vi "Multi-Channel ADC Viewer.vi"(0 "Channel Selection":T4, 1 "Start":bool, 5 "ADC Type":T1={"Channel Type"=enum."Single", "Resolution"=enum."8"}, 9 "Stop":bool, 11 "error in":errorcluster) -> (4 "Digital Waveform Graph":digitalwaveform(graph), 15 "error out":errorcluster)   [LabVIEW 2023]
doc: "This is simple ADC viewer which can plot the ADC data from the Analog to Digital conversion VI of different channels based on the user input, It can be a single channel viewer or a multi channel viewer. User can configure the resolution of the ADC. And also desired channels can be selected to view the ADC waveform."
uses:
  Type def/ChannelSelection.ctl
  Type def/ADCType.ctl
  Type def/ChannelType.ctl
  Type def/Resolution.ctl
  Type def/QueueOperations.ctl
  Type def/variant.ctl
  Type def/DataCluster.ctl
  Classes/Model Driver/Model Driver.lvclass
  Type def/U8ArrayCluster.ctl
panel:
  in  "Reset":bool
  # "MULTI-CHANNEL ADC VIEWER"
  # "INSTRUCTIONS\n\n1. Run the VI.\n2. Select the ADC Type -> Channel Type and Resolution.\n3. Channel Type can be -> Single Channel or 4-Channel.\n4. Resolution can be -> 2,4,8,12 or 16 bits.\n5. Use Channel selection option to view a particular channel\n    when using 4-Channel ADC.\n5. Press Start to start the ADC.\n6. Press Stop to stop the ADC.\n7. Press Reset to clear the Waveform Graph.\n8. Panel Close to Abort the VI."
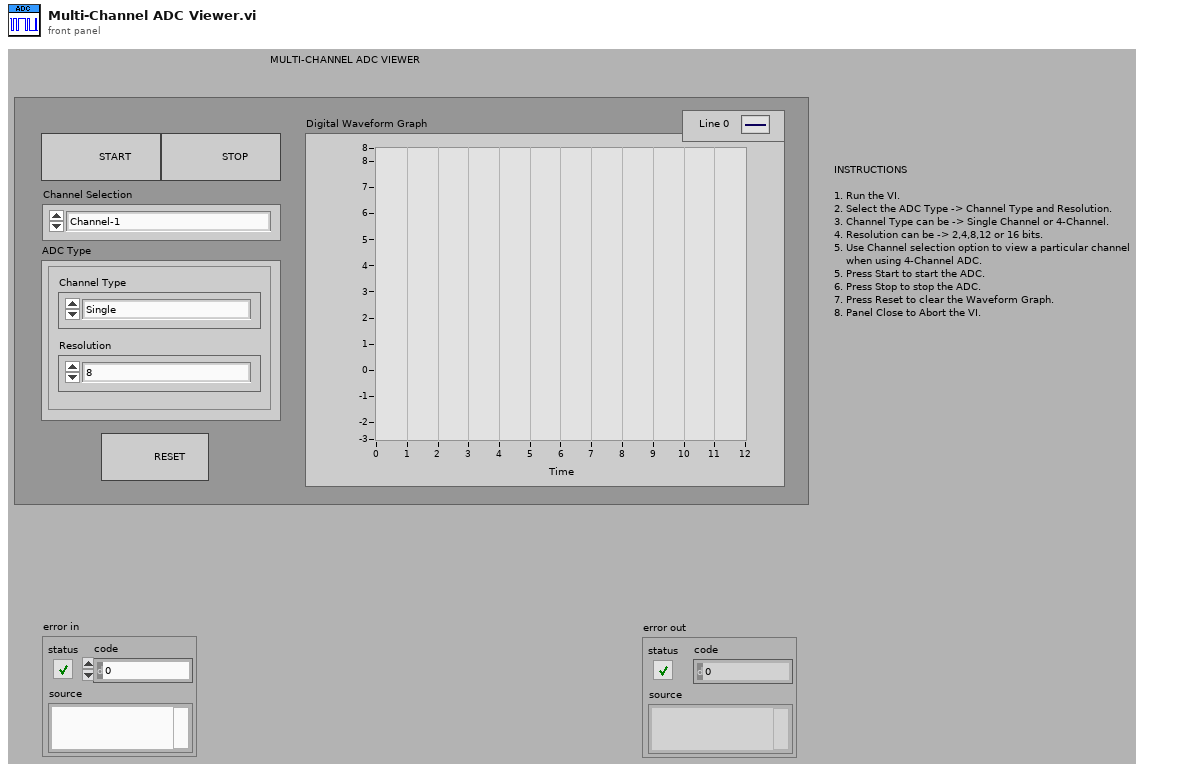
[diagram p1: front panel]
types:
  T1 = typedef "ADCType.ctl" = cluster{"Channel Type":T2, "Resolution":T3}
  T2 = typedef "ChannelType.ctl" = enum16{"Single", "4-Channel"}
  T3 = typedef "Resolution.ctl" = enum16{"2", "4", "8", "12", "16"}
  T4 = typedef "ChannelSelection.ctl" = enum16{"Channel-1", "Channel-2", "Channel-3", "Channel-4"}
  T5 = typedef "DataCluster.ctl" = cluster{"Stop":bool, "File Path":path, "Channel Selection":T4, "ADC Type":T1, "Digital Waveform Graph":digitalwaveform, "Start Time":dbl, "Elapsed Time":dbl, "Start":bool, "Model Driver Class":refnum<class "Model Driver.lvclass">, "Stop User Event":refnum<user-event>, "U8 Arrays":T6}
  T6 = typedef "U8ArrayCluster.ctl" = cluster{"Single Channel U8 array":u8[], "Mult Channel U8 array":u8[][], "1D Multi Channel U8 Array":u8[], "Channel 1 U8 Array":u8[], "Channel 2 U8 Array":u8[], "Channel 3 U8 Array":u8[], "Channel 4 U8 Array":u8[]}
  T7 = typedef "variant.ctl" = cluster{"Data":variant, "State":string}
  T8 = typedef "QueueOperations.ctl" = enum16{"Create", "Enqueue", "Enqueue N elements", "Dequeue", "Flush", "Release"}
  T9 = enum8{"Enabled", "Disabled", "Disabled and Grayed Out"}
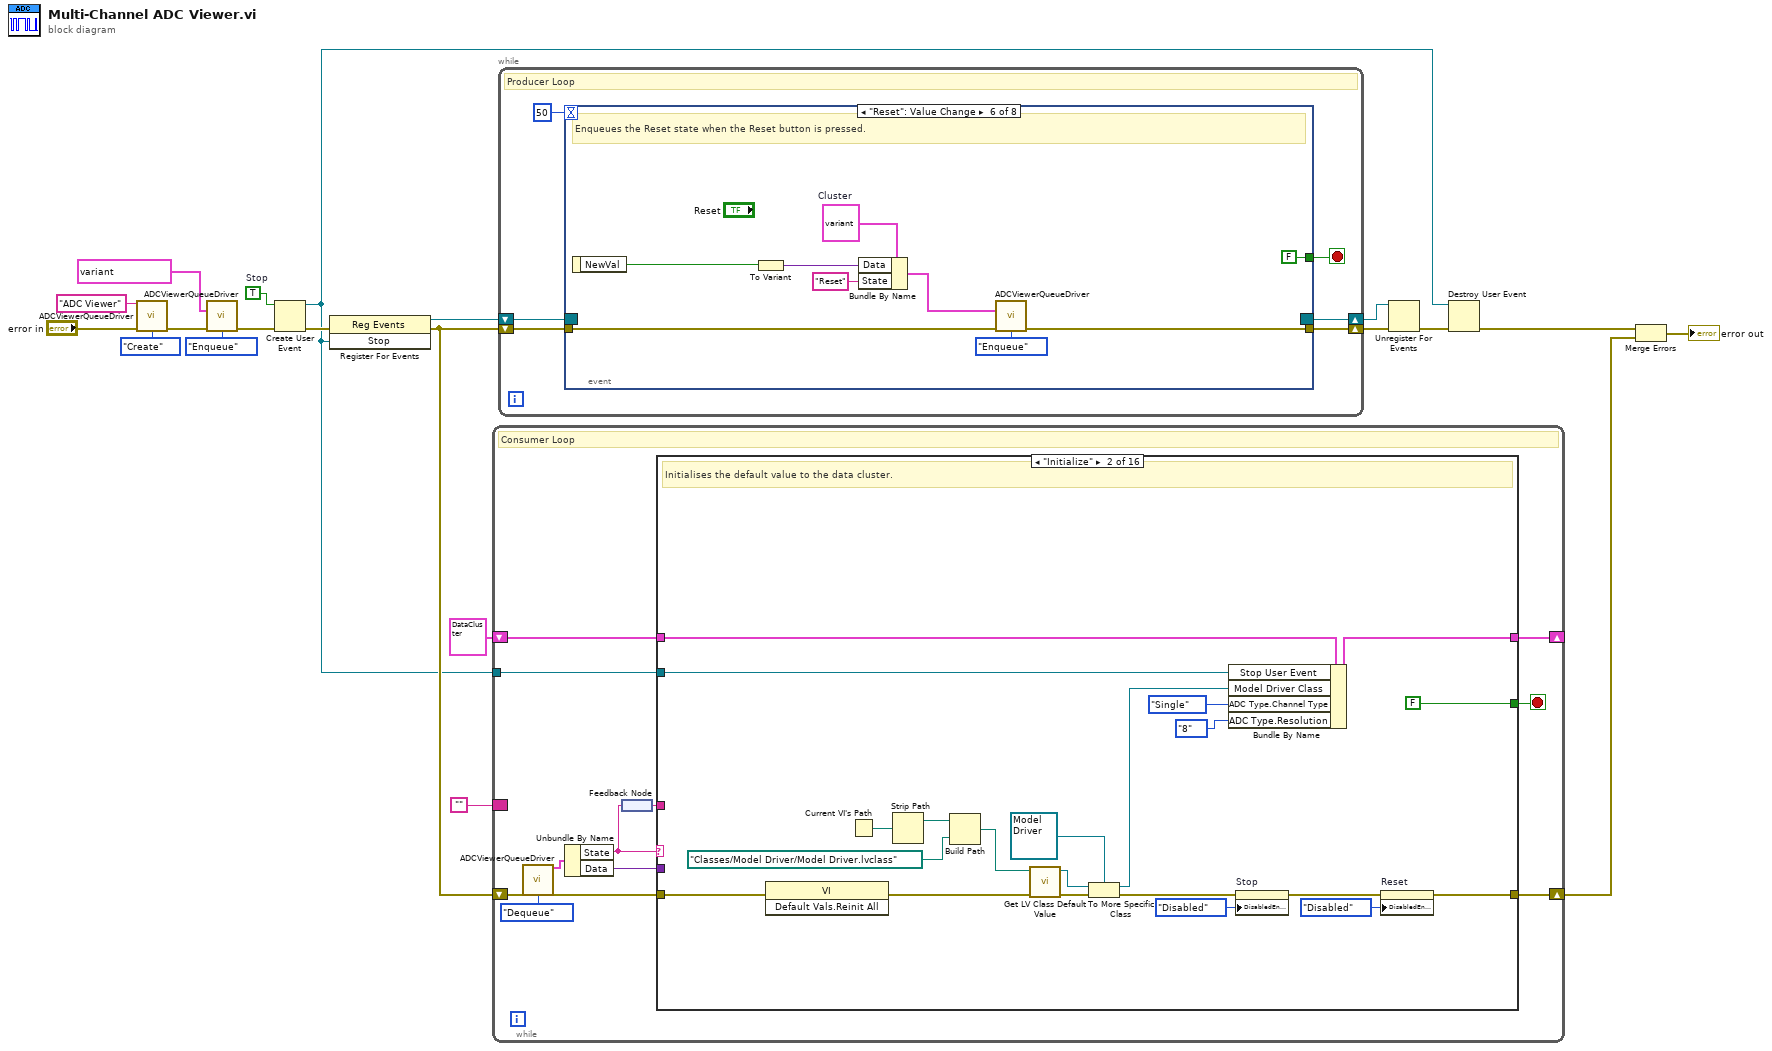
[diagram p0: block diagram]
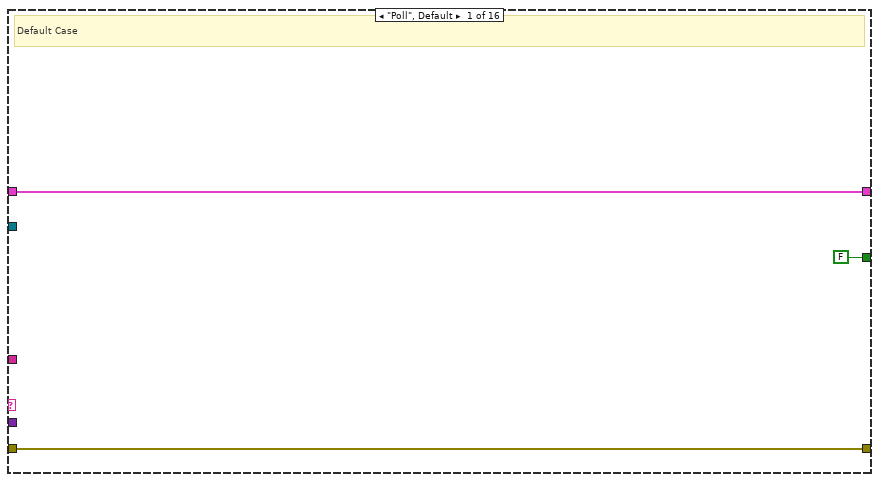
[diagram p2: hidden frame]
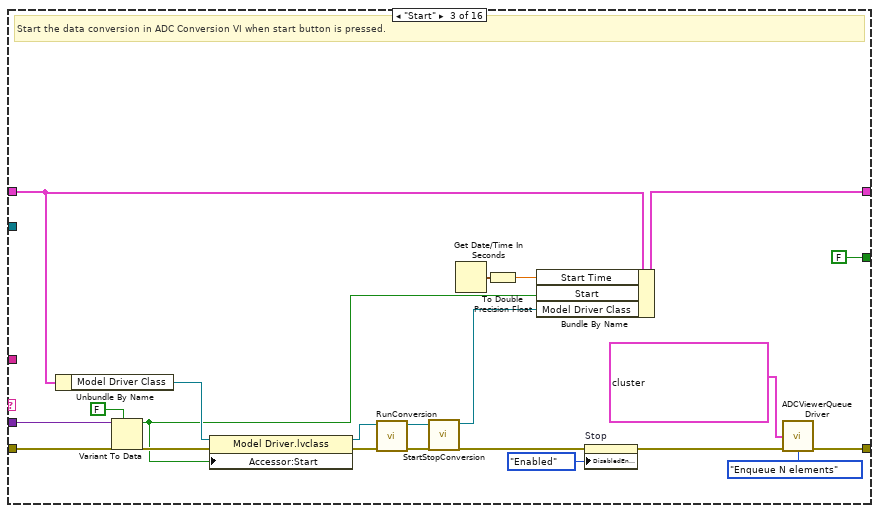
[diagram p3: hidden frame]
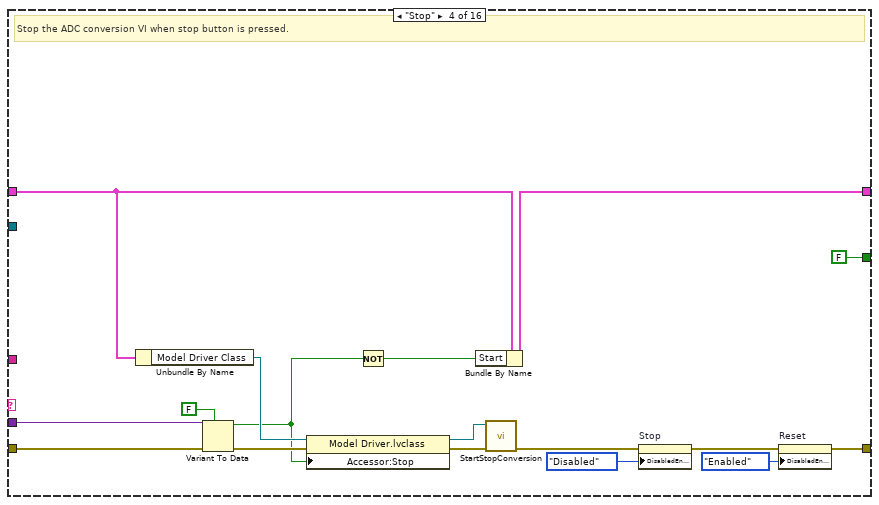
[diagram p4: hidden frame]
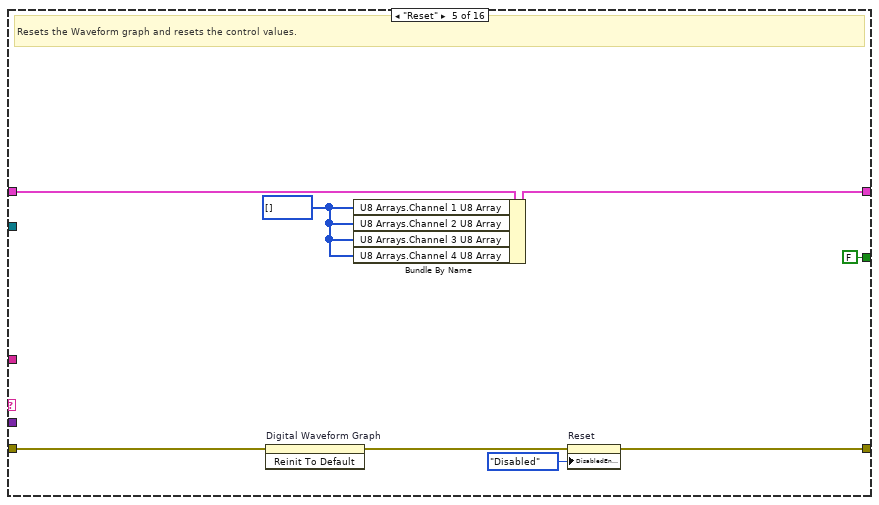
[diagram p5: hidden frame]
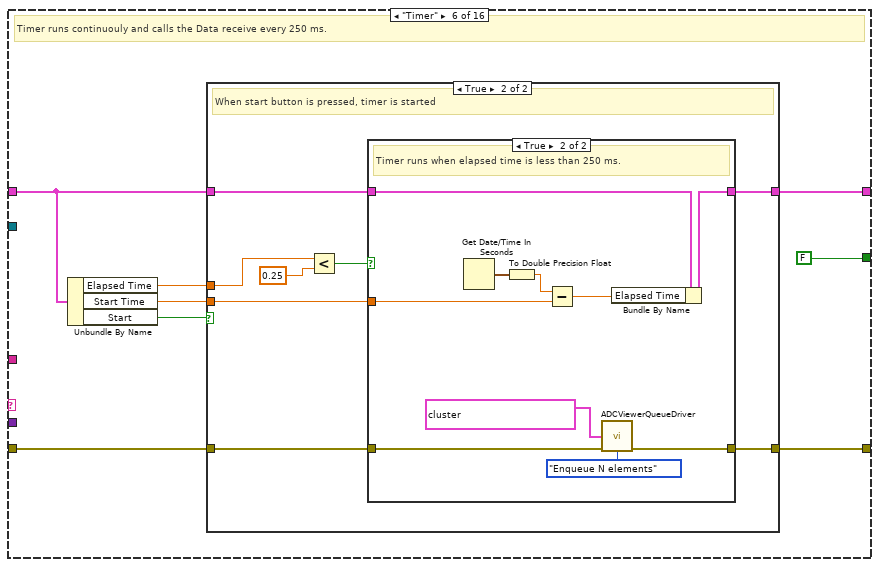
[diagram p6: hidden frame]
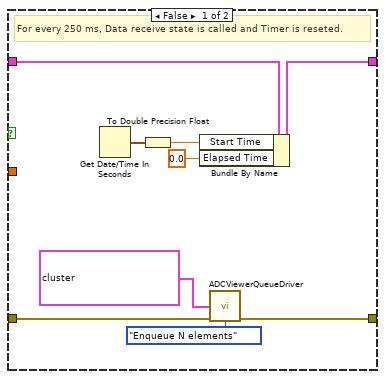
[diagram p8: hidden frame]
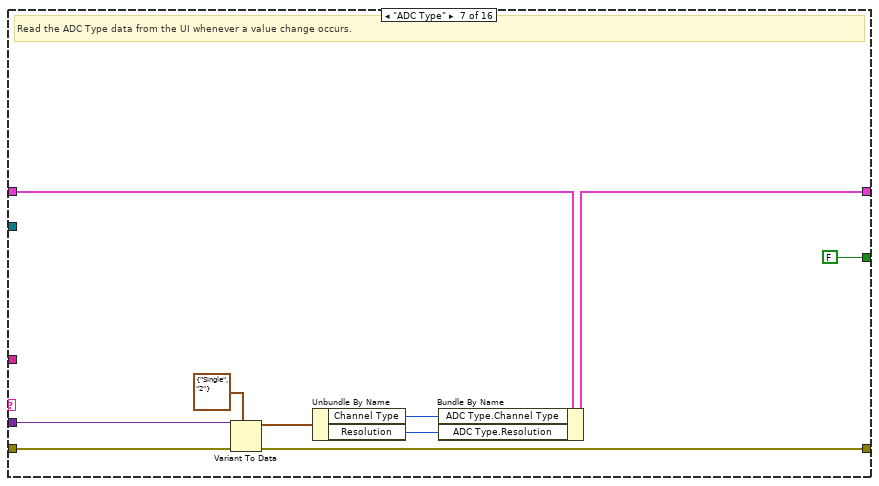
[diagram p9: hidden frame]
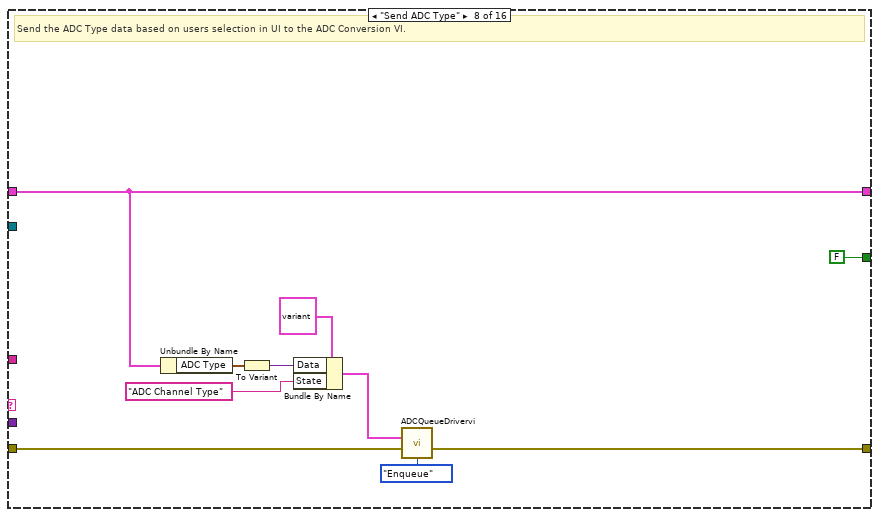
[diagram p10: hidden frame]
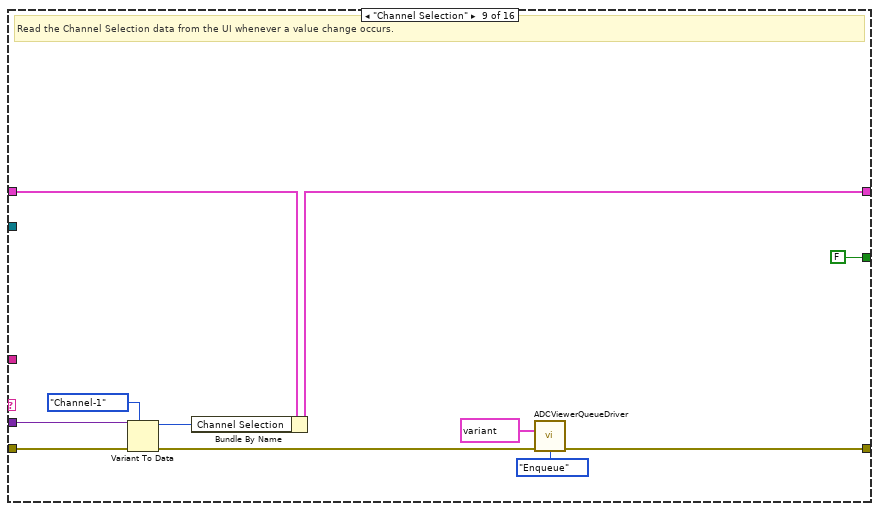
[diagram p11: hidden frame]
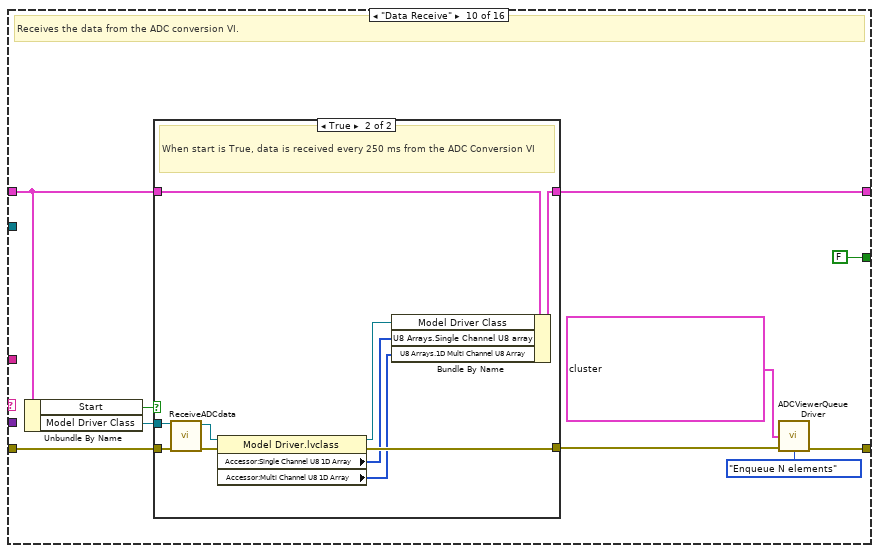
[diagram p12: hidden frame]
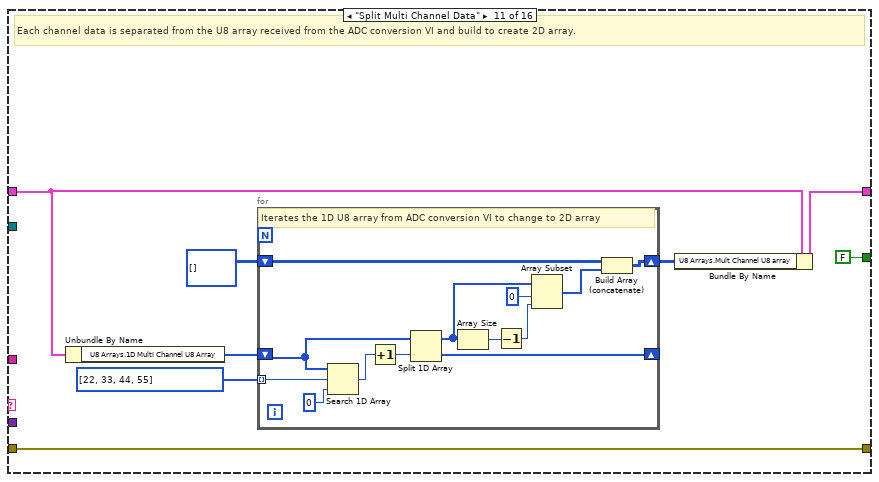
[diagram p14: hidden frame]
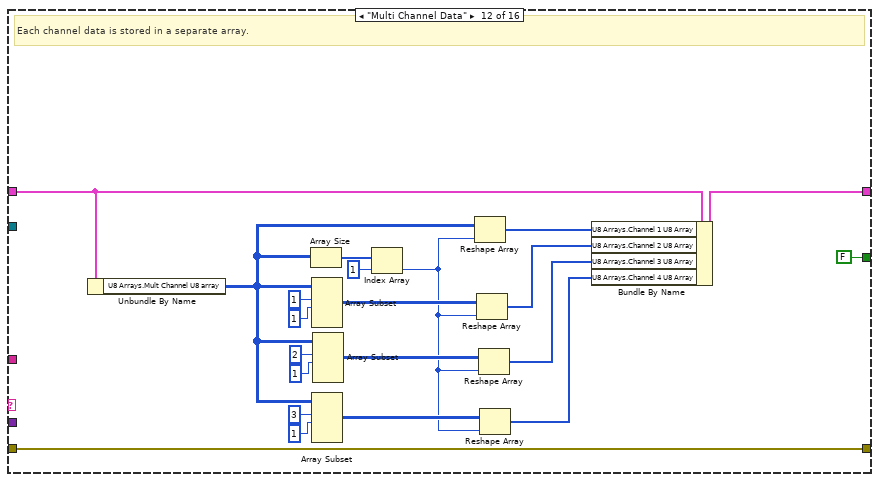
[diagram p15: hidden frame]
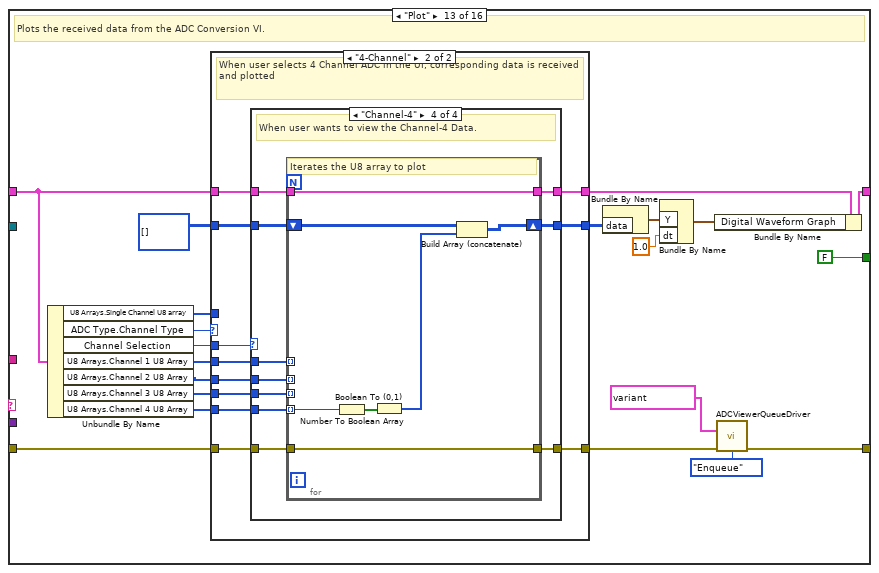
[diagram p16: hidden frame]
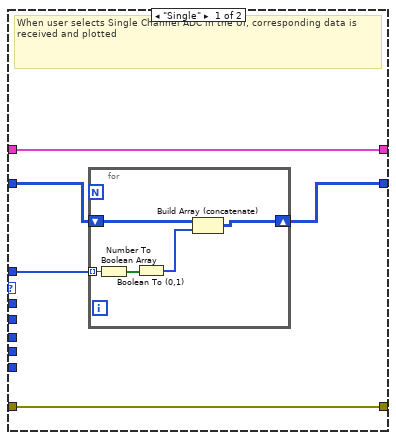
[diagram p17: hidden frame]
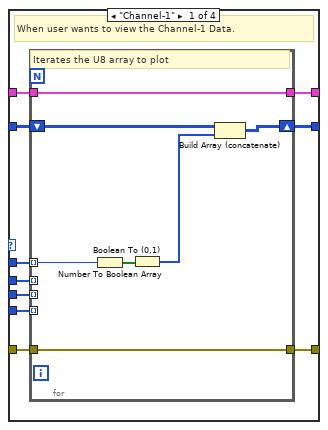
[diagram p18: hidden frame]
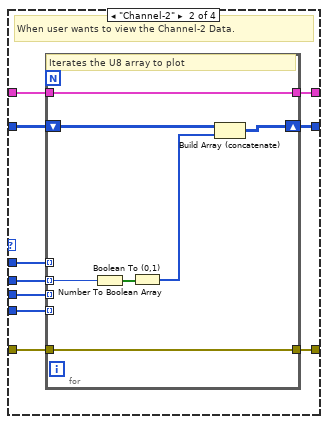
[diagram p19: hidden frame]
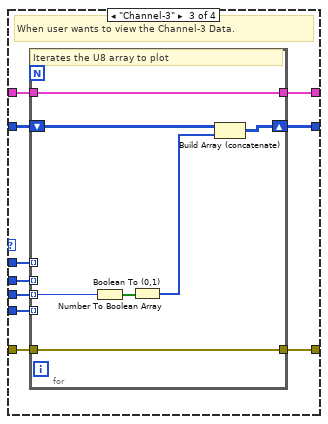
[diagram p20: hidden frame]
diagram:
  w8 = TRUE  # Stop
  n1 = call "ADCViewerQueueDriver.vi"("Queue Name"="ADC Viewer", "error in"="error in", "Queue Operations"=QueueOperations."Create") -> ("error out"=w19:errorcluster)  [unwired: 11 in, 1 out]
  n2 = call "ADCViewerQueueDriver.vi"("Enqueue State"=T7 {"Data"=variant, "State"="Initialize"}, "error in"=w19, "Queue Operations"=QueueOperations."Enqueue") -> ("error out"=w18:errorcluster)  [unwired: 11 in, 1 out]
  n3 = Create User Event(user event datatype=w8, error in=w18) -> (user event=w1:refnum<user-event>, error out=w9:errorcluster)
  n4 = register-events(error in=w9, w1) -> (reference out=w6:refnum<event-registration>, error out=w7:errorcluster)  [unwired: 1 in]
  n5 = while {
    shift-right: [w32] -> w13
    shift-left: w7 -> [w31]
    shift-right: [w24] -> _
    shift-left: T5 {"Stop"=FALSE, "File Path"=path "", "Channel Selection"=enum."Channel-1", "ADC Type"={"Channel Type"=enum."Single", "Resolution"=enum."2"}, "Digital Waveform Graph"={"t0"=timestamp(0 s since 1904-01-01), "dt"=0.0, "Y"={"transitions"=[], "data"=[]}}, "Start Time"=0.0, "Elapsed Time"=0.0, "Start"=FALSE, "Model Driver Class"=refnum, "Stop User Event"=refnum, "U8 Arrays"={"Single Channel U8 array"=[], "Mult Channel U8 array"=[], "1D Multi Channel U8 Array"=[], "Channel 1 U8 Array"=[], "Channel 2 U8 Array"=[], "Channel 3 U8 Array"=[], "Channel 4 U8 Array"=[]}} ("Cluster") -> [w25]
    border: "" -> [_]
    tunnel: w1 -> [w21]
    stop <- w26 stop-if-true
    # "Consumer Loop"
    n6 = call "ADCViewerQueueDriver.vi"("error in"=w31, "Queue Operations"=QueueOperations."Dequeue") -> ("Dequeue State"=w29:T7, "error out"=w30:errorcluster)  [unwired: 12 in]
    n7 = Unbundle By Name(w29) -> ("State"=w23:string, "Data"=w28:variant)
    n8 = feedback-in #1(w23) -> ()
    n9 = feedback #1() -> (w22:string)
    n10 = case shown="\"Initialize\"" w23 {
      tunnel: w30 -> [w33 w56 w75 w93 w97 w106 w150 w158 w171 w181 w201 w235 w248 w349 w363 w377]
      tunnel: [w33 w46 w70 w81 w100 w105 w141 w157 w162 w178 w201 w235 w238 w349 w353 w381] -> w32
      tunnel: w28 -> [_ _ w74 w92 _ _ w142 _ w167 _ _ _ _ _ _ _]
      tunnel: [FALSE FALSE FALSE FALSE FALSE FALSE FALSE FALSE FALSE FALSE FALSE FALSE FALSE FALSE FALSE TRUE] -> w26
      tunnel: w25 -> [w34 w54 w67 w89 w103 w110 w149 w156 w170 w175 w197 w234 w251 w347 w351 w383]
      tunnel: [w34 w50 w72 w91 w99 w109 w147 w156 w169 w179 w198 w219 w241 w347 w351 w383] -> w24
      tunnel: w22 -> [_ _ _ _ _ _ _ _ _ _ _ _ _ _ w362 _]
      tunnel: w21 -> [_ w47 _ _ _ _ _ _ _ _ _ _ _ _ _ _]
      frame "Poll", Default {
        # "Default Case"
      }
      frame "Initialize" {
        # "Initialises the default value to the data cluster."
        n11 = invoke class="VI" method="Default Vals.Reinit All"(error in=w56) -> (error out=w53:errorcluster)  [unwired: 2 in, 2 out]
        n12 = Current VI's Path() -> (path=w44:path)
        n13 = Strip Path(path=w44) -> (stripped path=w43:path)  [unwired: 1 out]
        n14 = Build Path(base path=w43, name or relative path=path "Classes/Model Driver/Model Driver.lvclass") -> (appended path=w41:path)
        n15 = call <vilib>:"Get LV Class Default Value.vi"("error in (no error)"=w53, "class path"=w41) -> ("error out"=w52:errorcluster, "object"=w51:refnum<class>)  [unwired: 8 in]
        n16 = To More Specific Class(target class=refnum<class "Model Driver.lvclass"> refnum ("Model Driver.lvclass"), reference=w51, error in=w52) -> (specific class reference=w48:refnum<class "Model Driver.lvclass">, error out=w37:errorcluster)
        n17 = Bundle By Name(cluster=w54, "Stop User Event"=w47, "Model Driver Class"=w48, "ADC Type.Channel Type"=ChannelType."Single", "ADC Type.Resolution"=Resolution."8") -> (w50:T5)
        n18 = property on="Stop" class="Bool"(error in=w37, "DisabledEnum"=T9."Disabled" ("Disabled")) -> (error out=w36:errorcluster)  [unwired: 1 in, 1 out]
        n19 = property on="Reset" class="Bool"(error in=w36, "DisabledEnum"=T9."Disabled" ("Disabled")) -> (error out=w46:errorcluster)  [unwired: 1 in, 1 out]
      }
      frame "Start" {
        # "Start the data conversion in ADC Conversion VI when start button is pressed."
        n20 = Unbundle By Name(w67) -> ("Model Driver Class"=w66:refnum<class "Model Driver.lvclass">)
        n21 = Variant To Data(error in=w75, type=FALSE, Variant=w74) -> (data=w65:bool, error out=w69:errorcluster)
        n22 = property class="Model Driver.lvclass"(reference=w66, error in=w69, "Accessor:Start"=w65) -> (reference out=w64:refnum<class "Model Driver.lvclass">, error out=w63:errorcluster)
        n23 = call "RunConversion.vi"("error in (no error)"=w63, "Model Driver in"=w64) -> ("error out"=w61:errorcluster, "Model Driver out"=w62:refnum<class "Model Driver.lvclass">)  [unwired: 8 in]
        n24 = call "StartStopConversion.vi"("error in (no error)"=w61, "Model Driver in"=w62) -> ("error out"=w59:errorcluster, "Model Driver out"=w57:refnum<class "Model Driver.lvclass">)  [unwired: 8 in]
        n25 = Get Date/Time In Seconds() -> (seconds since 1Jan1904=w77:timestamp)
        n26 = To Double Precision Float(number=w77) -> (double precision float=w76:dbl)
        n27 = Bundle By Name(cluster=w67, "Start Time"=w76, "Start"=w65, "Model Driver Class"=w57) -> (w72:T5)
        n28 = property on="Stop" class="Bool"(error in=w59, "DisabledEnum"=T9."Enabled" ("Disabled")) -> (error out=w58:errorcluster)  [unwired: 1 in, 1 out]
        n29 = call "ADCViewerQueueDriver.vi"("Array State"=T7[] [{"Data"=variant, "State"="Send ADC Type"}, {"Data"=variant, "State"="Timer"}], "error in"=w58, "Queue Operations"=QueueOperations."Enqueue N elements") -> ("error out"=w70:errorcluster)  [unwired: 11 in, 1 out]
      }
      frame "Stop" {
        # "Stop the ADC conversion VI when stop button is pressed."
        n30 = Unbundle By Name(w89) -> ("Model Driver Class"=w88:refnum<class "Model Driver.lvclass">)
        n31 = Variant To Data(error in=w93, type=FALSE, Variant=w92) -> (data=w85:bool, error out=w87:errorcluster)
        n32 = property class="Model Driver.lvclass"(reference=w88, error in=w87, "Accessor:Stop"=w85) -> (reference out=w84:refnum<class "Model Driver.lvclass">, error out=w86:errorcluster)
        n33 = Not(x=w85) -> (.not. x?=w90:bool)
        n34 = Bundle By Name(cluster=w89, "Start"=w90) -> (w91:T5)
        n35 = call "StartStopConversion.vi"("error in (no error)"=w86, "Model Driver in"=w84) -> ("error out"=w83:errorcluster)  [unwired: 8 in, 1 out]
        n36 = property on="Stop" class="Bool"(error in=w83, "DisabledEnum"=T9."Disabled" ("Disabled")) -> (error out=w82:errorcluster)  [unwired: 1 in, 1 out]
        n37 = property on="Reset" class="Bool"(error in=w82, "DisabledEnum"=T9."Enabled" ("Disabled")) -> (error out=w81:errorcluster)  [unwired: 1 in, 1 out]
      }
      frame "Reset" {
        w98 = u8[] [] ("U8 Arrays.Channel 1 U8 Array")
        # "Resets the Waveform graph and resets the control values."
        n38 = invoke on="Digital Waveform Graph" class="DigitalGraph (strict)" method="Reinit To Default"(error in=w97) -> (error out=w96:errorcluster)  [unwired: 2 in, 2 out]
        n39 = Bundle By Name(cluster=w103, "U8 Arrays.Channel 1 U8 Array"=w98, "U8 Arrays.Channel 2 U8 Array"=w98, "U8 Arrays.Channel 3 U8 Array"=w98, "U8 Arrays.Channel 4 U8 Array"=w98) -> (w99:T5)
        n40 = property on="Reset" class="Bool"(error in=w96, "DisabledEnum"=T9."Disabled" ("Disabled")) -> (error out=w100:errorcluster)  [unwired: 1 in, 1 out]
      }
      frame "Timer" {
        # "Timer runs continuouly and calls the Data receive every 250 ms."
        n41 = Unbundle By Name(w110) -> ("Elapsed Time"=w108:dbl, "Start Time"=w107:dbl, "Start"=w104:bool)
        n42 = case shown="True" w104 {
          tunnel: w110 -> [w113 w121]
          tunnel: [w113 w120] -> w109
          tunnel: w108 -> [_ w118]
          tunnel: w107 -> [_ w116]
          tunnel: w106 -> [w112 w115]
          tunnel: [w112 w114] -> w105
          frame False {
            # "When start button is not pressed."
          }
          frame True {
            # "When start button is pressed, timer is started"
            n43 = Less?(x=w118, y=0.25) -> (x < y?=w119:bool)
            n44 = case shown="True" w119 {
              tunnel: w121 -> [w130 w140]
              tunnel: [w129 w139] -> w120
              tunnel: w116 -> [_ w136]
              tunnel: w115 -> [w125 w134]
              tunnel: [w123 w133] -> w114
              frame False {
                # "For every 250 ms, Data receive state is called and Timer is reseted."
                n45 = Get Date/Time In Seconds() -> (seconds since 1Jan1904=w127:timestamp)
                n46 = To Double Precision Float(number=w127) -> (double precision float=w126:dbl)
                n47 = Bundle By Name(cluster=w130, "Start Time"=w126, "Elapsed Time"=0.0) -> (w129:T5)
                n48 = call "ADCViewerQueueDriver.vi"("Array State"=T7[] [{"Data"=variant, "State"="Timer"}, {"Data"=variant, "State"="Data Receive"}], "error in"=w125, "Queue Operations"=QueueOperations."Enqueue N elements") -> ("error out"=w123:errorcluster)  [unwired: 11 in, 1 out]
              }
              frame True {
                # "Timer runs when elapsed time is less than 250 ms."
                n49 = Get Date/Time In Seconds() -> (seconds since 1Jan1904=w138:timestamp)
                n50 = To Double Precision Float(number=w138) -> (double precision float=w137:dbl)
                n51 = Subtract(x=w137, y=w136) -> (x-y=w135:dbl)
                n52 = call "ADCViewerQueueDriver.vi"("Array State"=T7[] [{"Data"=variant, "State"="Timer"}, {"Data"=variant, "State"=""}], "error in"=w134, "Queue Operations"=QueueOperations."Enqueue N elements") -> ("error out"=w133:errorcluster)  [unwired: 11 in, 1 out]
                n53 = Bundle By Name(cluster=w140, "Elapsed Time"=w135) -> (w139:T5)
              }
            }
          }
        }
      }
      frame "ADC Type" {
        # "Read the ADC Type data from the UI whenever a value change occurs."
        n54 = Variant To Data(error in=w150, type=T1 {"Channel Type"=enum."Single", "Resolution"=enum."2"} ("NewVal"), Variant=w142) -> (data=w143:T1, error out=w141:errorcluster)
        n55 = Unbundle By Name(w143) -> ("Channel Type"=w146:T2, "Resolution"=w145:T3)
        n56 = Bundle By Name(cluster=w149, "ADC Type.Channel Type"=w146, "ADC Type.Resolution"=w145) -> (w147:T5)
      }
      frame "Send ADC Type" {
        # "Send the ADC Type data based on users selection in UI to the ADC Conversion VI."
        n57 = Unbundle By Name(w156) -> ("ADC Type"=w154:T1)
        n58 = To Variant(anything=w154) -> (Variant=w151:variant)
        n59 = Bundle By Name(cluster=T7 {"Data"=variant, "State"=""} ("Enqueue State"), "Data"=w151, "State"="ADC Channel Type") -> (w153:T7)
        n60 = call "ADCQueueDrivervi.vi"("Enqueue State"=w153, "error in"=w158, "Queue Operations"=QueueOperations."Enqueue") -> ("error out"=w157:errorcluster)  [unwired: 11 in, 1 out]
      }
      frame "Channel Selection" {
        # "Read the Channel Selection data from the UI whenever a value change occurs."
        n61 = Variant To Data(error in=w171, type=ChannelSelection."Channel-1" ("NewVal"), Variant=w167) -> (data=w165:T4, error out=w163:errorcluster)
        n62 = Bundle By Name(cluster=w170, "Channel Selection"=w165) -> (w169:T5)
        n63 = call "ADCViewerQueueDriver.vi"("Enqueue State"=T7 {"Data"=variant, "State"="Plot"}, "error in"=w163, "Queue Operations"=QueueOperations."Enqueue") -> ("error out"=w162:errorcluster)  [unwired: 11 in, 1 out]
      }
      frame "Data Receive" {
        # "Receives the data from the ADC conversion VI."
        n64 = Unbundle By Name(w175) -> ("Start"=w174:bool, "Model Driver Class"=w172:refnum<class "Model Driver.lvclass">)
        n65 = case shown="True" w174 {
          tunnel: w181 -> [w182 w191]
          tunnel: [w183 w193] -> w179
          tunnel: [w182 w189] -> w176
          tunnel: w175 -> [w183 w192]
          tunnel: w172 -> [_ w185]
          frame False {
            # "When Start is not pressed."
          }
          frame True {
            # "When start is True, data is received every 250 ms from the ADC Conversion VI"
            n66 = call "ReceiveADCdata.vi"("error in (no error)"=w191, "Model Driver in"=w185) -> ("error out"=w190:errorcluster, "Model Driver out"=w188:refnum<class "Model Driver.lvclass">)  [unwired: 8 in]
            n67 = property class="Model Driver.lvclass"(reference=w188, error in=w190) -> (reference out=w184:refnum<class "Model Driver.lvclass">, error out=w189:errorcluster, "Accessor:Single Channel U8 1D Array"=w187:u8[], "Accessor:Multi Channel U8 1D Array"=w186:u8[])
            n68 = Bundle By Name(cluster=w192, "Model Driver Class"=w184, "U8 Arrays.Single Channel U8 array"=w187, "U8 Arrays.1D Multi Channel U8 Array"=w186) -> (w193:T5)
          }
        }
        n69 = call "ADCViewerQueueDriver.vi"("Array State"=T7[] [{"Data"=variant, "State"="Split Multi Channel Data"}, {"Data"=variant, "State"="Multi Channel Data"}, {"Data"=variant, "State"="Plot"}], "error in"=w176, "Queue Operations"=QueueOperations."Enqueue N elements") -> ("error out"=w178:errorcluster)  [unwired: 11 in, 1 out]
      }
      frame "Split Multi Channel Data" {
        # "Each channel data is separated from the U8 array received from the ADC conversion VI and build to create 2D array."
        n70 = Unbundle By Name(w197) -> ("U8 Arrays.1D Multi Channel U8 Array"=w194:u8[])
        n71 = for {
          shift-right: [w204] -> _
          shift-left: w194 -> [w211]
          tunnel: u8[] [22, 33, 44, 55] ("array") -> [w210] mode=indexing
          shift-right: [w202] -> w196
          shift-left: u8[][] [] ("subarray") -> [w206]
          # "Iterates the 1D U8 array from ADC conversion VI to change to 2D array"
          n72 = Search 1D Array(1D array=w211, element=w210, start index (0)=0) -> (index of element=w213:i32)
          n73 = Increment(x=w213) -> (x+1=w212:i32)
          n74 = Split 1D Array(array=w211, index=w212) -> (first subarray=w205:u8[], second subarray=w204:u8[])
          n75 = Array Size(array=w205) -> (size(s)=w208:i32)
          n76 = Decrement(x=w208) -> (x-1=w207:i32)
          n77 = Array Subset(array=w205, index=0, length=w207) -> (w203:u8[])
          n78 = Build Array (concatenate)(w206, w203) -> (w202:u8[][])
        }
        n79 = Bundle By Name(cluster=w197, "U8 Arrays.Mult Channel U8 array"=w196) -> (w198:T5)
      }
      frame "Multi Channel Data" {
        # "Each channel data is stored in a separate array."
        n80 = Unbundle By Name(w234) -> ("U8 Arrays.Mult Channel U8 array"=w223:u8[][])
        n81 = Array Size(array=w223) -> (size(s)=w233:i32[])
        n82 = Array Subset(array=w223, index (row)=1 ("index"), length (row)=1 ("length")) -> (w229:u8[][])  [unwired: 2 in]
        n83 = Array Subset(array=w223, index (row)=3 ("index"), length (row)=1 ("length")) -> (w222:u8[][])  [unwired: 2 in]
        n84 = Array Subset(array=w223, index (row)=2 ("index"), length (row)=1 ("length")) -> (w226:u8[][])  [unwired: 2 in]
        n85 = Index Array(array=w233, index=1) -> (element=w221:i32)
        n86 = Reshape Array(w223, w221) -> (w218:u8[])
        n87 = Reshape Array(w229, w221) -> (w217:u8[])
        n88 = Reshape Array(w226, w221) -> (w216:u8[])
        n89 = Reshape Array(w222, w221) -> (w215:u8[])
        n90 = Bundle By Name(cluster=w234, "U8 Arrays.Channel 1 U8 Array"=w218, "U8 Arrays.Channel 2 U8 Array"=w217, "U8 Arrays.Channel 3 U8 Array"=w216, "U8 Arrays.Channel 4 U8 Array"=w215) -> (w219:T5)
      }
      frame "Plot" {
        # "Plots the received data from the ADC Conversion VI."
        n91 = Unbundle By Name(w251) -> ("U8 Arrays.Single Channel U8 array"=w253:u8[], "ADC Type.Channel Type"=w249:T2, "Channel Selection"=w247:T4, "U8 Arrays.Channel 1 U8 Array"=w246:u8[], "U8 Arrays.Channel 2 U8 Array"=w245:u8[], "U8 Arrays.Channel 3 U8 Array"=w244:u8[], "U8 Arrays.Channel 4 U8 Array"=w243:u8[])
        n92 = case shown="\"4-Channel\"" w249 {
          tunnel: i16[][] [] -> [w261 w272]
          tunnel: w253 -> [w260 _]
          tunnel: [w259 w277] -> w252
          tunnel: w251 -> [w258 w274]
          tunnel: [w258 w273] -> w250
          tunnel: w248 -> [w257 w276]
          tunnel: [w257 w275] -> w239
          tunnel: w247 -> [_ w271]
          tunnel: w246 -> [_ w270]
          tunnel: w245 -> [_ w269]
          tunnel: w244 -> [_ w268]
          tunnel: w243 -> [_ w267]
          frame "Single" {
            # "When user selects Single Channel ADC in the UI, corresponding data is received and plotted"
            n93 = for {
              tunnel: w260 -> [w266] mode=indexing
              shift-right: [w262] -> w259
              shift-left: w261 -> [w265]
              n94 = Number To Boolean Array(number=w266) -> (Boolean array=w263:bool[])
              n95 = Boolean To (0,1)(Boolean=w263) -> (0, 1=w264:i16[])
              n96 = Build Array (concatenate)(w265, w264) -> (w262:i16[][])
            }
          }
          frame "4-Channel" {
            # "When user selects 4 Channel ADC in the UI, corresponding data is received and plotted"
            n97 = case shown="\"Channel-4\"" w271 {
              tunnel: [w287 w304 w321 w338] -> w277
              tunnel: w276 -> [w286 w303 w320 w337]
              tunnel: [w285 w302 w319 w336] -> w275
              tunnel: w274 -> [w284 w301 w318 w335]
              tunnel: [w283 w300 w317 w334] -> w273
              tunnel: w272 -> [w282 w299 w316 w333]
              tunnel: w270 -> [w278 w295 w312 w329]
              tunnel: w269 -> [w281 w298 w315 w332]
              tunnel: w268 -> [w280 w297 w314 w331]
              tunnel: w267 -> [w279 w296 w313 w330]
              frame "Channel-1" {
                # "When user wants to view the Channel-1 Data."
                n98 = for {
                  shift-right: [w293] -> w287
                  shift-left: w282 -> [w294]
                  tunnel: w286 -> [w290]
                  tunnel: [w290] -> w285
                  tunnel: w284 -> [w289]
                  tunnel: [w289] -> w283
                  tunnel: w281 -> [_] mode=indexing
                  tunnel: w280 -> [_] mode=indexing
                  tunnel: w279 -> [_] mode=indexing
                  tunnel: w278 -> [w288] mode=indexing
                  # "Iterates the U8 array to plot"
                  n99 = Number To Boolean Array(number=w288) -> (Boolean array=w291:bool[])
                  n100 = Boolean To (0,1)(Boolean=w291) -> (0, 1=w292:i16[])
                  n101 = Build Array (concatenate)(w294, w292) -> (w293:i16[][])
                }
              }
              frame "Channel-2" {
                # "When user wants to view the Channel-2 Data."
                n102 = for {
                  shift-right: [w310] -> w304
                  shift-left: w299 -> [w311]
                  tunnel: w303 -> [w307]
                  tunnel: [w307] -> w302
                  tunnel: w301 -> [w306]
                  tunnel: [w306] -> w300
                  tunnel: w298 -> [w305] mode=indexing
                  tunnel: w297 -> [_] mode=indexing
                  tunnel: w296 -> [_] mode=indexing
                  tunnel: w295 -> [_] mode=indexing
                  # "Iterates the U8 array to plot"
                  n103 = Number To Boolean Array(number=w305) -> (Boolean array=w308:bool[])
                  n104 = Boolean To (0,1)(Boolean=w308) -> (0, 1=w309:i16[])
                  n105 = Build Array (concatenate)(w311, w309) -> (w310:i16[][])
                }
              }
              frame "Channel-3" {
                # "When user wants to view the Channel-3 Data."
                n106 = for {
                  shift-right: [w327] -> w321
                  shift-left: w316 -> [w328]
                  tunnel: w320 -> [w324]
                  tunnel: [w324] -> w319
                  tunnel: w318 -> [w323]
                  tunnel: [w323] -> w317
                  tunnel: w315 -> [_] mode=indexing
                  tunnel: w314 -> [w322] mode=indexing
                  tunnel: w313 -> [_] mode=indexing
                  tunnel: w312 -> [_] mode=indexing
                  # "Iterates the U8 array to plot"
                  n107 = Number To Boolean Array(number=w322) -> (Boolean array=w325:bool[])
                  n108 = Boolean To (0,1)(Boolean=w325) -> (0, 1=w326:i16[])
                  n109 = Build Array (concatenate)(w328, w326) -> (w327:i16[][])
                }
              }
              frame "Channel-4" {
                # "When user wants to view the Channel-4 Data."
                n110 = for {
                  shift-right: [w344] -> w338
                  shift-left: w333 -> [w345]
                  tunnel: w337 -> [w341]
                  tunnel: [w341] -> w336
                  tunnel: w335 -> [w340]
                  tunnel: [w340] -> w334
                  tunnel: w332 -> [_] mode=indexing
                  tunnel: w331 -> [_] mode=indexing
                  tunnel: w330 -> [w339] mode=indexing
                  tunnel: w329 -> [_] mode=indexing
                  # "Iterates the U8 array to plot"
                  n111 = Number To Boolean Array(number=w339) -> (Boolean array=w342:bool[])
                  n112 = Boolean To (0,1)(Boolean=w342) -> (0, 1=w343:i16[])
                  n113 = Build Array (concatenate)(w345, w343) -> (w344:i16[][])
                }
              }
            }
          }
        }
        n114 = Bundle By Name("data"=w252) -> (w242:digitaldata)  [unwired: 1 in]
        n115 = Bundle By Name("Y"=w242, "dt"=1.0) -> (w240:digitalwaveform)  [unwired: 1 in]
        n116 = Bundle By Name(cluster=w250, "Digital Waveform Graph"=w240) -> (w241:T5)
        n117 = call "ADCViewerQueueDriver.vi"("Enqueue State"=T7 {"Data"=variant, "State"="FP Update"}, "error in"=w239, "Queue Operations"=QueueOperations."Enqueue") -> ("error out"=w238:errorcluster)  [unwired: 11 in, 1 out]
      }
      frame "FP Update" {
        n118 = Unbundle By Name(w347) -> ("Digital Waveform Graph"=→"Digital Waveform Graph":digitalwaveform)
      }
      frame "Error" {
        # "Error Case"
        n119 = Unbundle By Name(w363) -> ("status"=w361:bool, "code"=w360:i32)
        n120 = call <vilib>:"Clear Errors.vi"("error in (no error)"=w363) -> ("error out"=w364:errorcluster)  [unwired: 5 in, 1 out]
        n121 = Format Into String(format string="Error occured at State : %s \nError Status : %s \nError Code : %d", initial string="", error in=w364, w362, w361, w360) -> (resulting string=w357:string, error out=w354:errorcluster)
        n122 = Unbundle By Name(w351) -> ("Stop User Event"=w350:refnum<user-event>)
        n123 = Two Button Dialog(message=w357, 1:"Exit" ("F button name (\"Cancel\")"), 2:"Continue" ("T button name (\"OK\")")) -> (T button?=w352:bool)
        n124 = case shown="True" w352 {
          tunnel: w354 -> [w366 w372]
          tunnel: [w366 w369] -> w353
          tunnel: w350 -> [_ w368]
          frame False {
            # "When user wishes to continue when an error occured."
          }
          frame True {
            # "When user wishes to exit when an error occured."
            n125 = call "ADCViewerQueueDriver.vi"("Enqueue State"=T7 {"Data"=variant, "State"="Exit"}, "error in"=w372, "Queue Operations"=QueueOperations."Enqueue") -> ("error out"=w371:errorcluster)  [unwired: 11 in, 1 out]
            n126 = Generate User Event(user event=w368, event data cluster=TRUE, error in=w371) -> (error out=w369:errorcluster)  [unwired: 1 in, 1 out]
          }
        }
      }
      frame "Exit" {
        # "Aborts this VI and ADC conversion VI."
        n127 = call "ADCViewerQueueDriver.vi"("error in"=w377, "Queue Operations"=QueueOperations."Flush") -> ("error out"=w375:errorcluster)  [unwired: 12 in, 1 out]
        n128 = call "ADCViewerQueueDriver.vi"("error in"=w375, "Queue Operations"=QueueOperations."Release") -> ("error out"=w374:errorcluster)  [unwired: 12 in, 1 out]
        n129 = call "ADCQueueDrivervi.vi"("Enqueue State"=T7 {"Data"=variant, "State"="Exit"}, "error in"=w374, "Queue Operations"=QueueOperations."Enqueue") -> ("error out"=w381:errorcluster)  [unwired: 11 in, 1 out]
      }
    }
  }
  n130 = while {
    shift-right: [w388] -> w14
    shift-left: w7 -> [w389]
    shift-right: [w384] -> w3
    shift-left: w6 -> [w385]
    stop <- w386 stop-if-true
    # "Producer Loop"
    n131 = event shown="[5] \"Reset\": Value Change" {
      selector: w385 -> [_ _ _ _ _ _ _ _]
      dyn-events: [_ _ _ _ _ _ _ _] -> w384
      timeout: 50 -> [_ _ _ _ _ _ _ _]
      tunnel: w389 -> [w391 w396 w409 w417 w421 w430 w438 w442]
      tunnel: [w391 w395 w408 w416 w420 w429 w438 w441] -> w388
      tunnel: [FALSE FALSE ("Discard?") FALSE ("Discard?") FALSE FALSE FALSE w437 w443] -> w386
      event Timeout {
        # "This event is triggered when no other event is triggered"
        n132 = event-data() -> ()  [unwired: 1 in, 1 out]
      }
      event Value Change {
        w400 = T7 {"Data"=variant, "State"=""}  # Cluster
        # "This event is triggered when the Channel is selected ."
        n133 = event-data() -> ("NewVal"=w394:T4)  [unwired: 1 in]
        n134 = To Variant(anything=w394) -> (Variant=w393:variant)
        n135 = Bundle By Name(cluster=w400, "Data"=w393, "State"="Channel Selection") -> (w399:T7)
        n136 = call "ADCViewerQueueDriver.vi"("Enqueue State"=w399, "error in"=w396, "Queue Operations"=QueueOperations."Enqueue") -> ("error out"=w395:errorcluster)  [unwired: 11 in, 1 out]
      }
      event Value Change {
        w407 = T7 {"Data"=variant, "State"=""}  # Cluster
        # "This event is triggered when the ADC Type is changed"
        n137 = event-data() -> ("NewVal"=w406:T1)  [unwired: 1 in]
        n138 = To Variant(anything=w406) -> (Variant=w405:variant)
        n139 = Bundle By Name(cluster=w407, "Data"=w405, "State"="ADC Type") -> (w404:T7)
        n140 = call "ADCViewerQueueDriver.vi"("Enqueue State"=w404, "error in"=w409, "Queue Operations"=QueueOperations."Enqueue") -> ("error out"=w408:errorcluster)  [unwired: 11 in, 1 out]
      }
      event "Start": Value Change {
        w414 = T7 {"Data"=variant, "State"=""}  # Cluster
        # "This event is triggered when the start button is pressed."
        n141 = event-data() -> ("NewVal"=w411:bool)  [unwired: 1 in]
        n142 = To Variant(anything=w411) -> (Variant=w413:variant)
        n143 = Bundle By Name(cluster=w414, "Data"=w413, "State"="Start") -> (w410:T7)
        n144 = call "ADCViewerQueueDriver.vi"("Enqueue State"=w410, "error in"=w417, "Queue Operations"=QueueOperations."Enqueue") -> ("error out"=w416:errorcluster)  [unwired: 11 in, 1 out]
      }
      event "Stop": Value Change {
        w425 = T7 {"Data"=variant, "State"=""}  # Cluster
        # "This event is triggered when the stop button is pressed."
        n145 = event-data() -> ("NewVal"=w419:bool)  [unwired: 1 in]
        n146 = To Variant(anything=w419) -> (Variant=w424:variant)
        n147 = Bundle By Name(cluster=w425, "Data"=w424, "State"="Stop") -> (w422:T7)
        n148 = call "ADCViewerQueueDriver.vi"("Enqueue State"=w422, "error in"=w421, "Queue Operations"=QueueOperations."Enqueue") -> ("error out"=w420:errorcluster)  [unwired: 11 in, 1 out]
      }
      event "Reset": Value Change {
        w434 = T7 {"Data"=variant, "State"=""}  # Cluster
        # "Enqueues the Reset state when the Reset button is pressed."
        n149 = event-data() -> ("NewVal"=w428:bool)  [unwired: 1 in]
        n150 = To Variant(anything=w428) -> (Variant=w433:variant)
        n151 = Bundle By Name(cluster=w434, "Data"=w433, "State"="Reset") -> (w431:T7)
        n152 = call "ADCViewerQueueDriver.vi"("Enqueue State"=w431, "error in"=w430, "Queue Operations"=QueueOperations."Enqueue") -> ("error out"=w429:errorcluster)  [unwired: 11 in, 1 out]
      }
      event User Event {
        # "This user event stops the Producer Loop."
        n153 = event-data() -> ("Stop"=w437:bool)  [unwired: 1 in]
      }
      event Panel Close? {
        w443 = TRUE ("Discard?")
        # "This event is triggered when the front panel of the UI is closed."
        n154 = event-data() -> ()  [unwired: 1 in, 1 out]
        n155 = call "ADCViewerQueueDriver.vi"("Enqueue State"=T7 {"Data"=variant, "State"="Exit"}, "error in"=w442, "Queue Operations"=QueueOperations."Enqueue") -> ("error out"=w441:errorcluster)  [unwired: 11 in, 1 out]
        n156 = event-data("Discard?"=w443) -> ()  [unwired: 1 in, 1 out]
      }
    }
  }
  n157 = Unregister For Events(event registration refnum=w3, error in=w14) -> (error out=w4:errorcluster)
  n158 = Destroy User Event(user event=w1, error in=w4) -> (error out=w5:errorcluster)
  n159 = Merge Errors(w5, w13) -> (→"error out":errorcluster)
